vi "Define.vi"(11 "Definition":T1) -> (3 "Text out":refnum<class "Text.lvclass">)   [LabVIEW 2020, in "Conditu2.lvlib" / "Columns.lvlib" / "Text.lvclass"]
uses:
  Text.lvclass
  C:/dev/lv20CE/lv-conditum-tools/Conditum-Clone/Columns/Type/Type.lvclass
  Text Definition.ctl
  Type/Definition.ctl
  Attributes.ctl
  Definition.ctl
  Field Type.ctl
  Type/Type.lvclass/Type.ctl
  Text.lvclass/Text.ctl
  Type/Type.lvclass
  Conditu2.lvlib
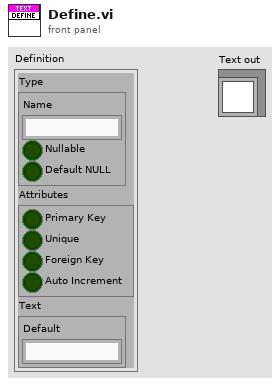
[diagram p1: front panel]
types:
  T1 = typedef "Conditu2.lvlib/Columns.lvlib/Text.lvclass/Text Definition.ctl" = cluster{"Type":T2, "Attributes":T3, "Text":T4}
  T2 = typedef "Conditu2.lvlib/Columns.lvlib/Type.lvclass/Definition.ctl" = cluster{"Name":string, "Nullable":bool, "Default NULL":bool}
  T3 = typedef "Conditu2.lvlib/Attributes.ctl" = cluster{"Primary Key":bool, "Unique":bool, "Foreign Key":bool, "Auto Increment":bool}
  T4 = typedef "Conditu2.lvlib/Columns.lvlib/Text.lvclass/Definition.ctl" = cluster{"Default":string}
  T5 = typedef "Conditu2.lvlib/Field Type.ctl" = enum16{"None", "ID", "Boolean", "Integer", "Double", "Timestamp", "String", "Text", "Entity"}
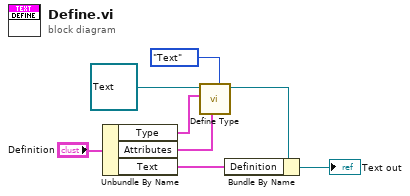
[diagram p0: block diagram]
diagram:
  n1 = Unbundle By Name("Definition") -> ("Type"=w6:T2, "Attributes"=w2:T3, "Text"=w5:T4)
  n2 = call "Define Type.vi"("Type"=Field_Type."Text", "Attributes"=w2, "Definition"=w6, "Type in"=refnum<class "Text.lvclass"> refnum ("Text out")) -> ("Type out"=w4:refnum<class "Text.lvclass">)  [unwired: 7 in]
  n3 = Bundle By Name(cluster=w4, "Definition"=w5) -> (→"Text out":refnum<class "Text.lvclass">)
